vi "Parse Query String.vi"(11 "query string":string) -> (3 "Variant":variant)   [LabVIEW 2020, in "Netatmo-WeatherStation.lvlib"]
uses:
  Netatmo-WeatherStation.lvlib
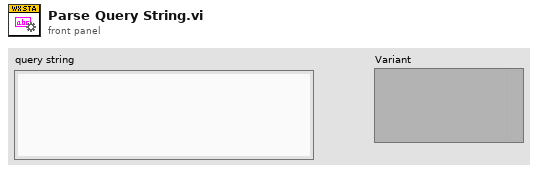
[diagram p1: front panel]
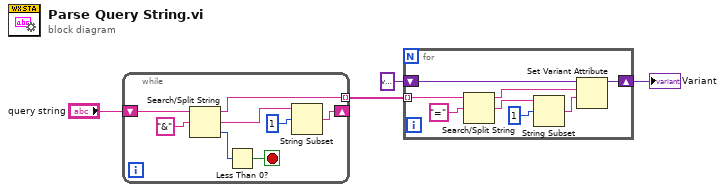
[diagram p0: block diagram]
diagram:
  n1 = while {
    shift-right: [w7] -> _
    shift-left: "query string" -> [w12]
    tunnel: [w10] -> w3 mode=indexing
    stop <- w6 stop-if-true
    n2 = Search/Split String(string=w12, search string/char (-)="&") -> (substring before match=w10:string, match + rest of string=w9:string, offset of match=w5:i32)  [unwired: 1 in]
    n3 = Less Than 0?(x=w5) -> (x < 0?=w6:bool)
    n4 = String Subset(string=w9, offset (0)=1) -> (substring=w7:string)  [unwired: 1 in]
  }
  n5 = for {
    tunnel: w3 -> [w19] mode=indexing
    shift-right: [w13] -> w1
    shift-left: variant ("map") -> [w16]
    n6 = Search/Split String(string=w19, search string/char (-)="=") -> (substring before match=w15:string, match + rest of string=w18:string)  [unwired: 1 in, 1 out]
    n7 = String Subset(string=w18, offset (0)=1) -> (substring=w14:string)  [unwired: 1 in]
    n8 = Set Variant Attribute(Variant=w16, name=w15, value=w14) -> (Variant out=w13:variant)  [unwired: 1 in, 2 out]
  }
  "Variant" <- w1
